vi "testIsTelQueueFromDdsFull.vi"(8 "error in (no error)":errorcluster) -> (0 "error out":errorcluster)   [LabVIEW 2018]
doc: "Test the IsTcpClientQueueFull.vi with queueFromDds option."
uses:
  src/TcpServer/TcpServer.lvclass
  src/TcpServerTel/typedef/enqueueOptionsTypeDef.ctl
  src/TcpServer/TcpServer.lvclass/TcpServer.ctl
  src/TcpServerTel/TcpServerTel.lvclass/TcpServerTel.ctl
  <vilib>/addons/_JKI Toolkits/Caraya/classes/Assert/Assert False.vi
  <vilib>/addons/_JKI Toolkits/Caraya/classes/Assert/Assert True.vi
  src/TcpServerTel/TcpServerTel.lvclass
  <vilib>/addons/_JKI Toolkits/Caraya/classes/Test/Test.lvclass
  <vilib>/addons/_JKI Toolkits/Caraya/classes/Assert/Assert.lvclass
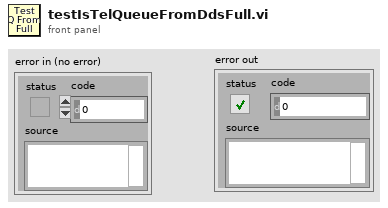
[diagram p1: front panel]
types:
  T1 = typedef "TcpServerTel.lvclass/enqueueOptionsTypeDef.ctl" = enum16{"lossy enqueue", "normal enqueue"}
  T2 = cluster{"cmdServerPort":u16, "telServerPort":u16, "serverTimeout (ms)":i32, "serverBytesToRead":i32, "maxSizeQueueTel":i32, "EnqueueOptions":T1, "timeoutQueueTel (ms)":i32, "tcpClientQueueMaxSize":i32, "timeoutInMs":i32}
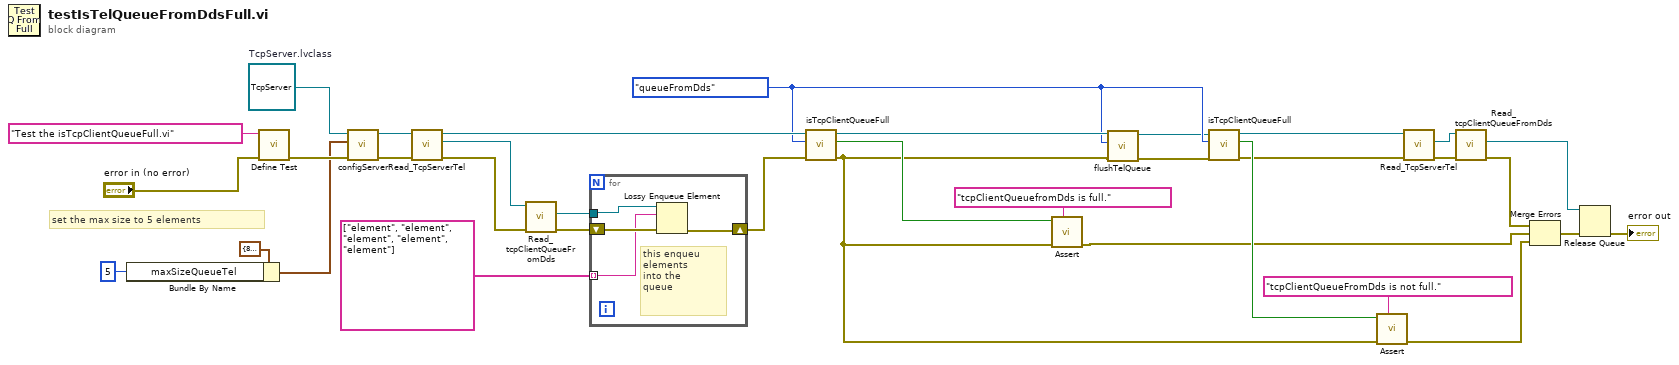
[diagram p0: block diagram]
diagram:
  w6 = enum16{"queueFromDds", "queueToDds"}."queueFromDds" ("queueName")
  w24 = refnum<class "TcpServer.lvclass"> refnum  # TcpServer.lvclass
  # "set the max size to 5 elements"
  n1 = Bundle By Name(cluster=T2 {"cmdServerPort"=8888, "telServerPort"=8889, "serverTimeout (ms)"=100, "serverBytesToRead"=32768, "maxSizeQueueTel"=1000, "EnqueueOptions"=enum."lossy enqueue", "timeoutQueueTel (ms)"=50, "tcpClientQueueMaxSize"=1000, "timeoutInMs"=100} ("ServerConfiguration"), "maxSizeQueueTel"=5 ("telQueueServerMaxSize")) -> (w2:T2)
  n2 = call <vilib>:"Define Test.vi"("error in (no error)"="error in (no error)", "Label (VI Title)"="Test the isTcpClientQueueFull.vi") -> ("error out"=w23:errorcluster)  [unwired: 9 in]
  n3 = call "configServer.vi"("error in (no error)"=w23, "ServerConfiguration"=w2, "tcpServer in"=w24) -> ("error out"=w11:errorcluster, "tcpServer out"=w12:refnum<class "TcpServer.lvclass">)  [unwired: 7 in]
  n4 = call "Read_TcpServerTel.vi"("error in (no error)"=w11, "TcpServer in"=w12) -> ("error out"=w10:errorcluster, "TcpServerTel.lvclass"=w9:refnum<class "TcpServerTel.lvclass">, "TcpServer out"=w8:refnum<class "TcpServer.lvclass">)  [unwired: 7 in]
  n5 = call "Read_tcpClientQueueFromDds.vi"("error in (no error)"=w10, "TcpServerTel in"=w9) -> ("error out"=w14:errorcluster, "tcpClientQueueFromDds"=w13:refnum<queue>)  [unwired: 7 in, 1 out]
  n6 = for {
    shift-right: [w38] -> w7
    shift-left: w14 -> [w39]
    tunnel: string[] ["element", "element", "element", "element", "element"] -> [w36] mode=indexing
    tunnel: w13 -> [w37]
    # "this enqueu\nelements\ninto the\nqueue"
    n7 = Lossy Enqueue Element(queue=w37, element=w36, error in (no error)=w39) -> (error out=w38:errorcluster)  [unwired: 3 out]
  }
  n8 = call "isTcpClientQueueFull.vi"("error in (no error)"=w7, "queueName"=w6, "tcpServer in"=w8) -> ("error out"=w4:errorcluster, "queueFull"=w30:bool, "tcpServer out"=w22:refnum<class "TcpServer.lvclass">)  [unwired: 6 in]
  n9 = call-poly <vilib>:"Assert.vi"("Label"="tcpClientQueuefromDds is full.", "error in (no error)"=w4, "True?"=w30) -> ("error out"=w17:errorcluster)  [unwired: 8 in]
  n10 = call "flushTelQueue.vi"("error in (no error)"=w4, "queueName"=w6, "TcpServer in"=w22) -> ("error out"=w3:errorcluster, "TcpServer out"=w5:refnum<class "TcpServer.lvclass">)  [unwired: 6 in, 1 out]
  n11 = call "isTcpClientQueueFull.vi"("error in (no error)"=w3, "queueName"=w6, "tcpServer in"=w5) -> ("error out"=w18:errorcluster, "queueFull"=w20:bool, "tcpServer out"=w19:refnum<class "TcpServer.lvclass">)  [unwired: 6 in]
  n12 = call-poly <vilib>:"Assert.vi"("Label"="tcpClientQueueFromDds is not full.", "error in (no error)"=w4, "False?"=w20) -> ("error out"=w16:errorcluster)  [unwired: 8 in]
  n13 = call "Read_TcpServerTel.vi"("error in (no error)"=w18, "TcpServer in"=w19) -> ("error out"=w29:errorcluster, "TcpServerTel.lvclass"=w28:refnum<class "TcpServerTel.lvclass">)  [unwired: 7 in, 1 out]
  n14 = call "Read_tcpClientQueueFromDds.vi"("error in (no error)"=w29, "TcpServerTel in"=w28) -> ("error out"=w26:errorcluster, "tcpClientQueueFromDds"=w27:refnum<queue>)  [unwired: 7 in, 1 out]
  n15 = Merge Errors(w26, w17, w16) -> (w31:errorcluster)
  n16 = Release Queue(queue=w27, error in (no error)=w31) -> (error out=→"error out":errorcluster)  [unwired: 1 in, 2 out]
